vi "Rec.vi"(3 "N":dbl, 5 "t":dbl, 6 "Граница":dbl, 7 "Temper":dbl, 8 "Пересчет":dbl[](array[numeric]), 9 "Вип":dbl[](array[numeric]), 10 "Atm":dbl[](array[numeric]), 11 "Время":dbl[](array[numeric])) -> (0 "n":dbl, 1 "DT":dbl, 2 "раз":dbl, 4 "time":dbl)   [LabVIEW 2018]
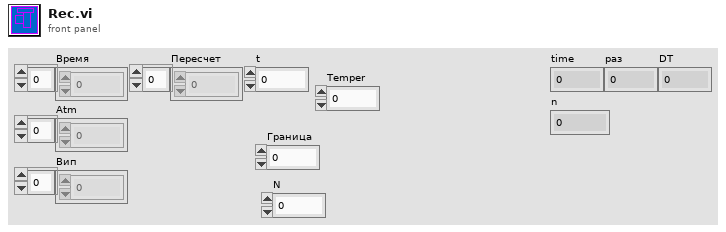
[diagram p1: front panel]
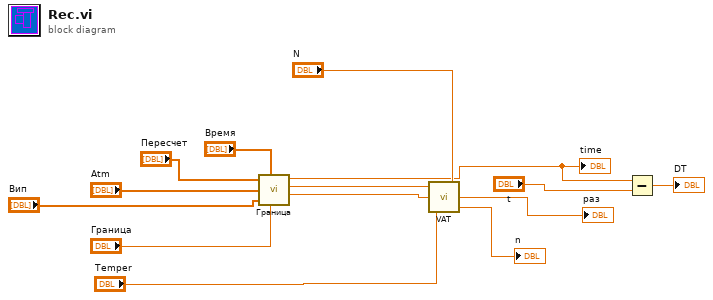
[diagram p0: block diagram]
diagram:
  n1 = call "Граница.vi"("Перерасчет"="Пересчет", "Time"="Время", "Atm"="Atm", "Вип"="Вип", "Граница"="Граница") -> ("time"=w2:dbl, "Вип"=w8:dbl, "Atm"=w7:dbl)  [unwired: 1 out]
  "time" <- w2
  n2 = call "VAT.vi"("Разность"="N", "Temper"="Temper", "Атмосферное"=w7, "Вип"=w8) -> ("n"=→"n":dbl, "раз"=→"раз":dbl)
  n3 = Subtract(x=w2, y="t") -> (x-y=→"DT":dbl)
